vi "HW_Poll_Tracker_1x.vi"(8 "error in":errorcluster, 11 "VISA resource name in":refnum<visa-resource-name>="ASRL3::INSTR") -> (0 "error out":errorcluster, 1 "Read buffer":string, 2 "Parameters output":T1, 3 "VISA resource name out":refnum<visa-resource-name>)   [LabVIEW 2016]
panel:
  out "Sensors response":string
  out "Port data status":i32
  out "Port data status index":i32
  out "FPS status":i32
  out "Poll records":u32
  out "FPS target index":i32
  out "Matrix mode status":string
  out "Matrix mode index":i32
  out "Coordinate mode status":string
  out "Coordinate mode index":i32
  out "Binary mode status":string
  out "Binary mode index":i32
  out "Array of tokens":string[](array[string])
  out "token index":i32
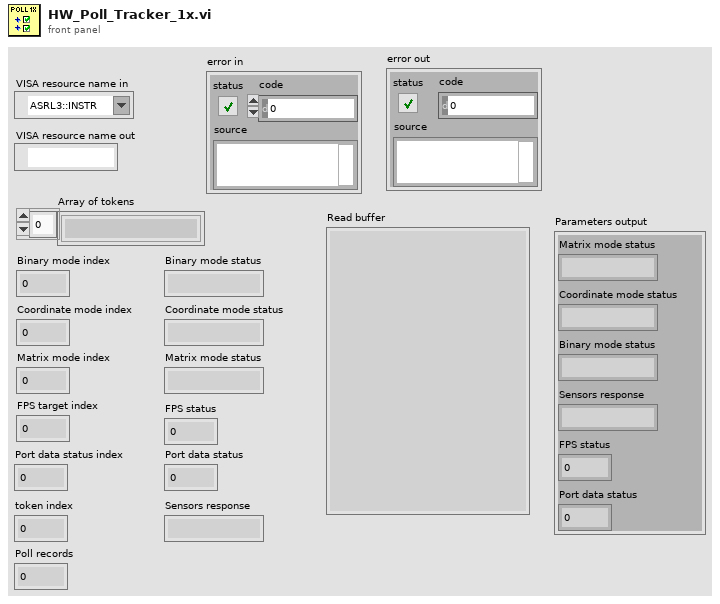
[diagram p1: front panel]
types:
  T1 = cluster{"Matrix mode status":string, "Coordinate mode status":string, "Binary mode status":string, "Sensors response":string, "FPS status":i32, "Port data status":i32}
  T2 = cluster{"token string":string, "token string":string, "token string":string, "trimmed string":string, i32, i32}
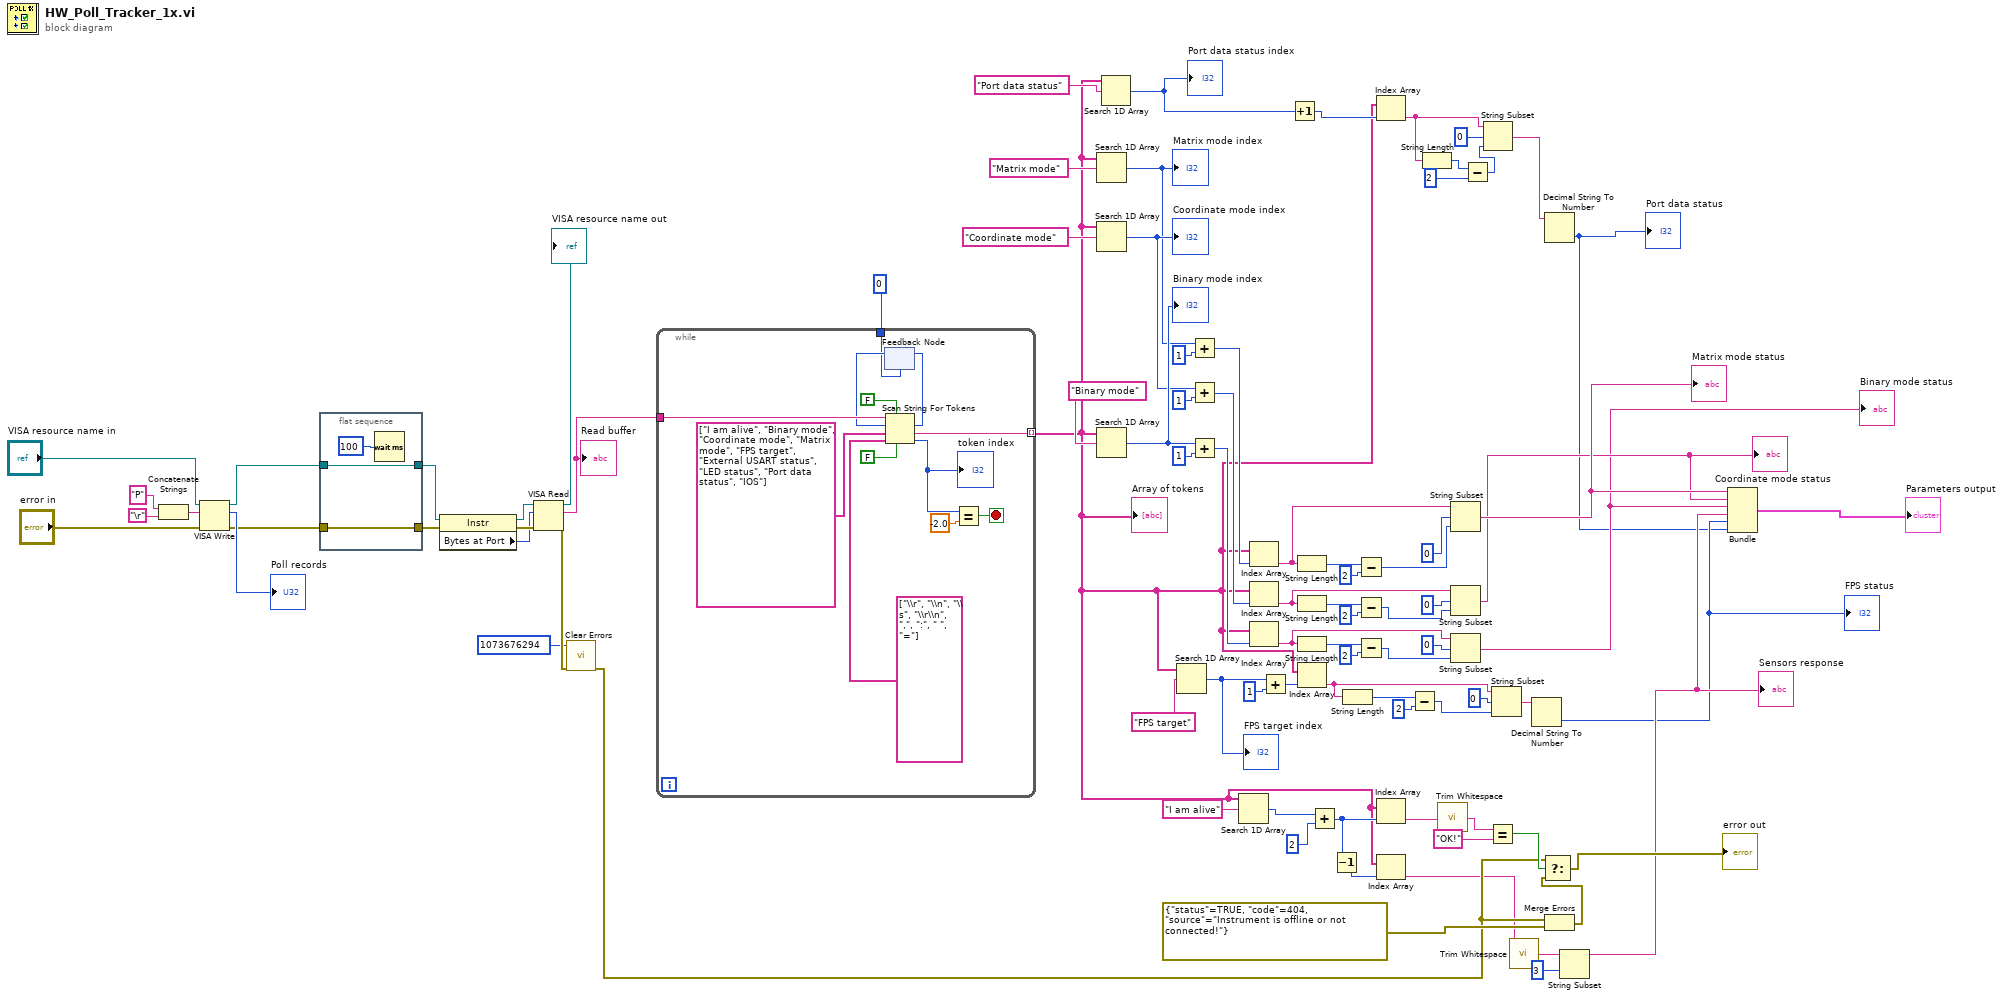
[diagram p0: block diagram]
diagram:
  n1 = Concatenate Strings("P" ("write buffer"), "\r") -> (w86:string)
  n2 = VISA Write(VISA resource name="VISA resource name in", write buffer=w86, error in (no error)="error in") -> (VISA resource name out=w61:refnum<visa-resource-name>, return count=→"Poll records":u32, error out=w59:errorcluster)
  n3 = flat-sequence {
    tunnel: [w90] -> w62
    tunnel: w61 -> [w90]
    tunnel: [w89] -> w60
    tunnel: w59 -> [w89]
    frame #0 {
      n4 = Wait (ms)(milliseconds to wait=u32 100) -> ()  [unwired: 1 out]
    }
  }
  n5 = property class="Instr"(reference=w62, error in=w60) -> (reference out=w84:refnum<visa-resource-name>, error out=w83:errorcluster, "Bytes at Port"=w82:u32)
  n6 = VISA Read(VISA resource name=w84, byte count=w82, error in (no error)=w83) -> (VISA resource name out=→"VISA resource name out":refnum<visa-resource-name>, read buffer=w81:string, error out=w17:errorcluster)  [unwired: 1 out]
  "Read buffer" <- w81
  n7 = call <vilib>:"Clear Errors.vi"("error in (no error)"=w17, "specific error code to clear (0: all)"=1073676294) -> ("error out"=w16:errorcluster)  [unwired: 4 in, 1 out]
  n8 = while {
    tunnel: w81 -> [w103]
    tunnel: [w93] -> w13 mode=indexing
    tunnel: 0 ("offset past token") -> [w92]
    stop <- w99 stop-if-true
    n9 = feedback #1(w92) -> (w100:i32)
    n10 = Scan String For Tokens(4:FALSE ("use cached delim/oper data? (F)"), 5:FALSE ("allow empty tokens? (F)"), 6:string[] ["\\r", "\\n", "\\s", "\\r\\n", ",", ":", " ", "="] ("delimiters"), 7:string[] ["I am alive", "Binary mode", "Coordinate mode", "Matrix mode", "FPS target", "External USART status", "LED status", "Port data status", "IOS"] ("Tokens"), 8:w100, 9:w103) -> (0:w97:i32, 1:w93:string, 2:w101:i32)  [unwired: 1 out]
    "token index" <- w97
    n11 = feedback-in #1(w101) -> ()
    n12 = Equal?(x=w97, y=-2.0) -> (x = y?=w99:bool)
  }
  "Array of tokens" <- w13
  n13 = Search 1D Array(1D array=w13, element="Matrix mode") -> (index of element=w70:i32)  [unwired: 1 in]
  "Matrix mode index" <- w70
  n14 = Search 1D Array(1D array=w13, element="Coordinate mode") -> (index of element=w74:i32)  [unwired: 1 in]
  "Coordinate mode index" <- w74
  n15 = Search 1D Array(1D array=w13, element="Binary mode") -> (index of element=w78:i32)  [unwired: 1 in]
  "Binary mode index" <- w78
  n16 = Search 1D Array(1D array=w13, element="Port data status") -> (index of element=w35:i32)  [unwired: 1 in]
  "Port data status index" <- w35
  n17 = Search 1D Array(1D array=w13, element="FPS target") -> (index of element=w66:i32)  [unwired: 1 in]
  "FPS target index" <- w66
  n18 = Add(x=w70, y=1) -> (x+y=w71:i32)
  n19 = Add(x=w74, y=1) -> (x+y=w75:i32)
  n20 = Add(x=w78, y=1) -> (x+y=w79:i32)
  n21 = Search 1D Array(1D array=w13, element="I am alive") -> (index of element=w26:i32)  [unwired: 1 in]
  n22 = Index Array(array=w13, index=w71) -> (element=w39:string)
  n23 = Index Array(array=w13, index=w75) -> (element=w37:string)
  n24 = Index Array(array=w13, index=w79) -> (element=w56:string)
  n25 = Add(x=w66, y=1) -> (x+y=w67:i32)
  n26 = Increment(x=w35) -> (x+1=w34:i32)
  n27 = String Length(string=w39) -> (length=w51:i32)
  n28 = String Length(string=w37) -> (length=w42:i32)
  n29 = String Length(string=w56) -> (length=w55:i32)
  n30 = Index Array(array=w13, index=w67) -> (element=w38:string)
  n31 = Add(x=w26, y=2) -> (x+y=w14:i32)
  n32 = Decrement(x=w14) -> (x-1=w12:i32)
  n33 = String Length(string=w38) -> (length=w47:i32)
  n34 = Subtract(x=w51, y=2) -> (x-y=w49:i32)
  n35 = Subtract(x=w42, y=2) -> (x-y=w40:i32)
  n36 = Subtract(x=w55, y=2) -> (x-y=w53:i32)
  n37 = Index Array(array=w13, index=w34) -> (element=w33:string)
  n38 = Index Array(array=w13, index=w14) -> (element=w24:string)
  n39 = Index Array(array=w13, index=w12) -> (element=w11:string)
  n40 = Subtract(x=w47, y=2) -> (x-y=w45:i32)
  n41 = String Length(string=w33) -> (length=w32:i32)
  n42 = call <vilib>:"Trim Whitespace.vi"("string"=w24) -> ("trimmed string"=w23:string)  [unwired: 1 in]
  n43 = String Subset(string=w39, offset (0)=0, length (rest)=w49) -> (substring=w7:string)
  "Matrix mode status" <- w7
  n44 = String Subset(string=w37, offset (0)=0, length (rest)=w40) -> (substring=w6:string)
  "Coordinate mode status" <- w6
  n45 = String Subset(string=w56, offset (0)=0, length (rest)=w53) -> (substring=w5:string)
  "Binary mode status" <- w5
  n46 = Subtract(x=w32, y=2) -> (x-y=w30:i32)
  n47 = String Subset(string=w33, offset (0)=0, length (rest)=w30) -> (substring=w28:string)
  n48 = Equal?(x=w23, y="OK!") -> (x = y?=w21:bool)
  n49 = String Subset(string=w38, offset (0)=0, length (rest)=w45) -> (substring=w44:string)
  n50 = call <vilib>:"Trim Whitespace.vi"("string"=w11) -> ("trimmed string"=w10:string)  [unwired: 1 in]
  n51 = Decimal String To Number(string=w44) -> (number=w3:i32)  [unwired: 2 in, 1 out]
  "FPS status" <- w3
  n52 = Decimal String To Number(string=w28) -> (number=w2:i32)  [unwired: 2 in, 1 out]
  "Port data status" <- w2
  n53 = Merge Errors(w16, errorcluster {"status"=TRUE, "code"=404, "source"="Instrument is offline or not connected!"} ("error in")) -> (w19:errorcluster)
  n54 = Select(t=w16, s=w21, f=w19) -> (s? t:f=→"error out":errorcluster)
  n55 = String Subset(string=w10, offset (0)=3) -> (substring=w4:string)  [unwired: 1 in]
  "Sensors response" <- w4
  n56 = Bundle("token string"=w7, "token string"=w6, "token string"=w5, "trimmed string"=w4, w3, w2) -> (→"Parameters output":T2)  [unwired: 1 in]
